vi "Get WorksheetPart.vi"(8 "error in":errorcluster, 10 "Sheet Name":string, 11 "SpreadsheetDoc in":refnum<k24>) -> (0 "error out":errorcluster, 2 "WorksheetPart":refnum<k24>, 3 "SpreadsheetDoc out":refnum<k24>, 5 "SheetName":string)   [LabVIEW 2019, in "Open Xml.lvlib"]
uses:
  Open Xml.lvlib
  D:/git/Open-Xml-LabVIEW/Source/DocumentFormat.OpenXml.dll
  DocumentFormat.OpenXml.dll
  D:/git/Open-Xml-LabVIEW/Source/DocumentFormat.OpenXml.Framework.dll
  DocumentFormat.OpenXml.Framework.dll
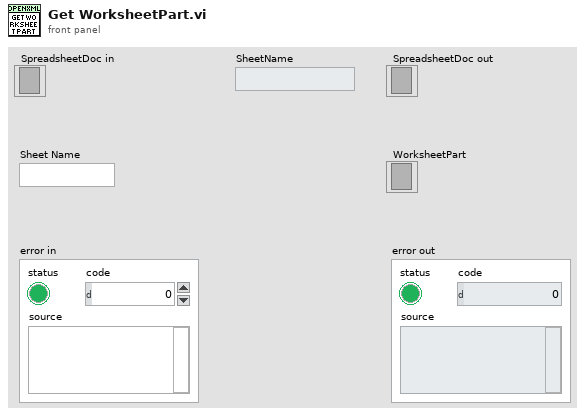
[diagram p1: front panel]
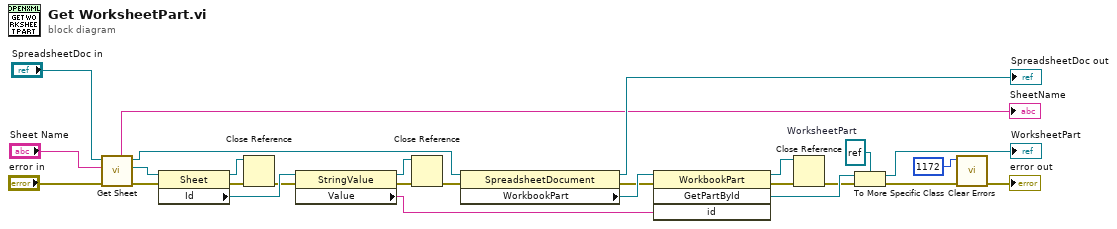
[diagram p0: block diagram]
diagram:
  w9 = refnum<k24> refnum  # WorksheetPart
  n1 = call "Get Sheet.vi"("error in"="error in", "SheetName"="Sheet Name", "SpreadsheetDoc in"="SpreadsheetDoc in") -> ("error out"=w18:errorcluster, "Sheet"=w17:refnum<k24>, "SpreadsheetDoc out"=w24:refnum<k24>, "SheetName"=→"SheetName":string)  [unwired: 4 in, 1 out]
  n2 = property class="Sheet"(reference=w17, error in=w18) -> (reference out=w12:refnum<k24>, error out=w19:errorcluster, "Id"=w20:refnum<k24>)
  n3 = Close Reference(reference=w12, error in (no error)=w19) -> (error out=w13:errorcluster)
  n4 = property class="StringValue"(reference=w20, error in=w13) -> (reference out=w6:refnum<k24>, error out=w15:errorcluster, "Value"=w16:string)
  n5 = Close Reference(reference=w6, error in (no error)=w15) -> (error out=w7:errorcluster)
  n6 = property class="SpreadsheetDocument"(reference=w24, error in=w7) -> (reference out=→"SpreadsheetDoc out":refnum<k24>, error out=w22:errorcluster, "WorkbookPart"=w23:refnum<k24>)
  n7 = invoke class="WorkbookPart" method="GetPartById"(reference=w23, error in=w22, "id"=w16) -> (reference out=w4:refnum<k24>, error out=w21:errorcluster, "GetPartById"=w10:refnum<k24>)  [unwired: 1 in, 1 out]
  n8 = Close Reference(reference=w4, error in (no error)=w21) -> (error out=w5:errorcluster)
  n9 = To More Specific Class(target class=w9, reference=w10, error in=w5) -> (specific class reference=→"WorksheetPart":refnum<k24>, error out=w11:errorcluster)
  n10 = call <vilib>:"Clear Errors.vi"("error in (no error)"=w11, "specific error code to clear (0: all)"=1172) -> ("error out"=→"error out":errorcluster)  [unwired: 4 in, 1 out]
